vi "FTW-CodeGen-GenerateCode.vi"(0 "State In":T2, 5 "XRef":refnum<vi>, 7 "Terms":T1(array[cluster]), 9 "Diagram":refnum<vi>) -> (4 "State Out":T2, 6 "Reply":string[](array[string]), 8 "Generated Code?":bool)   [LabVIEW 2013, in "Featherweight.lvlib" / "FTW-SQLite-Fetch.xnode"]
uses:
  FTW-SQLite-Fetch.xnode
  FTW-CodeGen-State.ctl
  FTW-CodeGen.lvlib
  Featherweight.lvlib
panel:
  # "Inputs"
  # "Outputs"
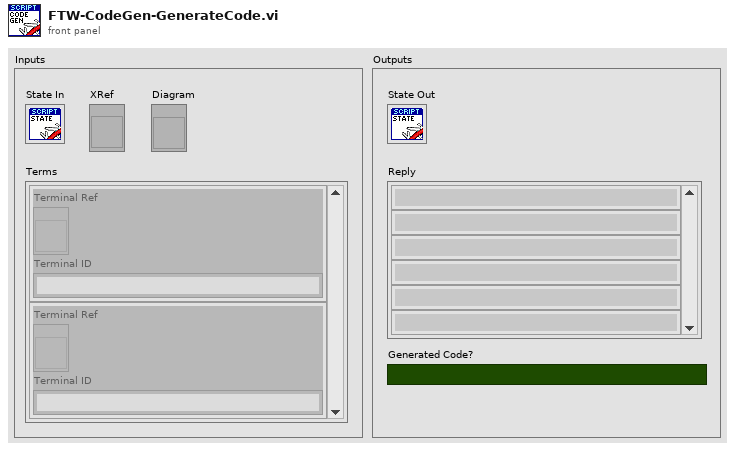
[diagram p1: front panel]
types:
  T1 = cluster{"Terminal Ref":refnum<vi>, "Terminal ID":string}[]
  T2 = typedef "Featherweight.lvlib/FTW-SQLite-Fetch.xnode/FTW-CodeGen-State.ctl" = cluster{"Dummy":string}
  T3 = typedef "LVPositionTypeDef.ctl" = cluster{"Left":i32, "Top":i32}
  T4 = typedef "Featherweight.lvlib/FTW-Reflection-Types.ctl" = enum16{"Unknown", "Void", "Array", "Cluster", "LVObject", "Boolean", "I8", "I16", "I32", "I64", "U8", "U16", "U32", "U64", "SGL", "DBL", "EXT", "CSG", "CDB", "CXT", "FXP", "EnumU8", "EnumU16", "EnumU32", "EnumU64", "SGLwithUnit", "DBLwithUnit", "EXTwithUnit", "CSGwithUnit", "CDBwithUnit", "CXTwithUnit", "String", "Path", "Picture", "Tag", "LVVariant", "Timestamp", "WaveformI8", "WaveformI16", "WaveformI32", "WaveformI64", "WaveformU8", "WaveformU16", "WaveformU32", "WaveformU64", "WaveformSGL", "WaveformDBL", "WaveformEXT", "WaveformCSG", "WaveformCDB", "WaveformCXT", "WaveformDigital", "WaveformUnknownType", "DigitalData", "DynamicData", "ExternalData", "FileByteStream", "TDMStream", "dotNET", "ActiveX", "VIServerReference", "VIReference", "ApplicationInstance", "Menu", "ConnectionDataSocket", "ConnectionVISA", "ConnectionBluetooth", "ConnectionIrDA", "ConnectionTCP", "ConnectionUDP", "ConnectionHTTPClient", "ConnectionFTP", "Occurrence", "Notifier", "Queue", "Rendezvous", "Semaphore", "RTFIFO", "EventPublisher", "EventRegistration", "EventCallback", "DataValueReference", "GenericClass", "GenericClassTag", "GenericClassDeepCopy", "GenericClassFlattened", "GenericClassTagFlattened", "GenericReferenceType", "WindowsRegistry", "OverloadedDatalogRef", "ReferenceUnknownType"}
  T5 = cluster{"Element Name":string, "Element Type":T4, "Element Value":variant}[]
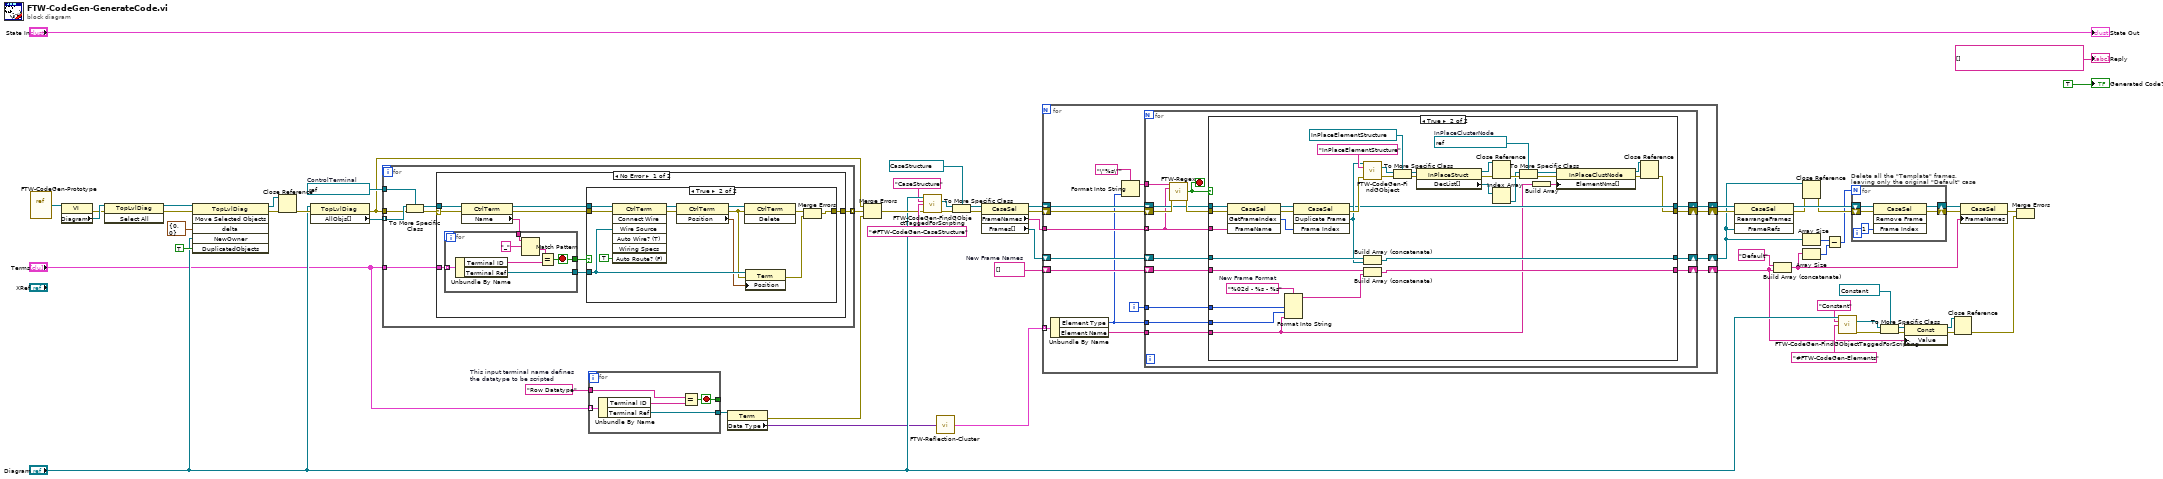
[diagram p0: block diagram]
diagram:
  w19 = string[] []  # New Frame Names
  w38 = "Row Datatype"  # This input terminal name defines the datatype to be scripted
  w57 = refnum<vi> refnum  # ControlTerminal
  n1 = vi-ref "FTW-CodeGen-Prototype.vi"() -> (w50:refnum<vi>)
  n2 = property class="VI"(reference=w50) -> (error out=w49:errorcluster, "Diagram"=w56:refnum<vi>)  [unwired: 1 in, 1 out]
  n3 = invoke class="TopLvlDiag" method="Select All"(reference=w56, error in=w49) -> (reference out=w60:refnum<vi>, error out=w59:errorcluster)  [unwired: 1 in, 1 out]
  n4 = invoke class="TopLvlDiag" method="Move Selected Objects"(reference=w60, error in=w59, "delta"=cluster{"X":i32, "Y":i32} {"X"=0, "Y"=0} ("X/Y Delta"), "NewOwner"="Diagram", "DuplicatedObjects"=TRUE ("Duplicate? (F)")) -> (reference out=w46:refnum<vi>, error out=w48:errorcluster)  [unwired: 1 in, 4 out]
  n5 = Close Reference(reference=w46, error in (no error)=w48) -> (error out=w47:errorcluster)
  n6 = property class="TopLvlDiag"(reference="Diagram", error in=w47) -> (error out=w54:errorcluster, "AllObjs[]"=w58:refnum<vi>[])  [unwired: 1 out]
  n7 = for {
    tunnel: w58 -> [w69] mode=indexing
    tunnel: w54 -> [w68]
    tunnel: w57 -> [w67]
    tunnel: "Terms" -> [w64]
    tunnel: [w63] -> w55 mode=indexing
    n8 = To More Specific Class(target class=w67, reference=w69, error in=w68) -> (specific class reference=w65:refnum<vi>, error out=w66:errorcluster)
    n9 = case shown="No Error" w66 {
      selector: w66 -> [w77 _]
      tunnel: w65 -> [w78 _]
      tunnel: w64 -> [w76 _]
      tunnel: [w71 _] -> w63
      frame No Error {
        n10 = property class="CtrlTerm"(reference=w78, error in=w77) -> (reference out=w73:refnum<vi>, error out=w72:errorcluster, "Name"=w75:string)
        n11 = for {
          tunnel: w76 -> [w98] mode=indexing
          tunnel: w75 -> [w96]
          tunnel: [w97] -> w74
          tunnel: [w92] -> w70
          stop <- w92 stop-if-true
          n12 = Unbundle By Name(w98) -> ("Terminal ID"=w93:string, "Terminal Ref"=w97:refnum<vi>)
          n13 = Match Pattern(string=w96, regular expression="_") -> (after substring=w94:string)  [unwired: 1 in, 3 out]
          n14 = Equal?(x=w94, y=w93) -> (x = y?=w92:bool)
        }
        n15 = case shown="True" w70 {
          tunnel: w74 -> [_ w83]
          tunnel: w73 -> [_ w91]
          tunnel: w72 -> [w79 w90]
          tunnel: [w79 w85] -> w71
          frame False {
          }
          frame True {
            n16 = invoke class="CtrlTerm" method="Connect Wire"(reference=w91, error in=w90, "Wire Source"=w83, "Auto Route? (F)"=TRUE) -> (reference out=w89:refnum<vi>, error out=w87:errorcluster)  [unwired: 3 in, 5 out]
            n17 = property class="CtrlTerm"(reference=w89, error in=w87) -> (reference out=w88:refnum<vi>, error out=w82:errorcluster, "Position"=w80:T3)
            n18 = invoke class="CtrlTerm" method="Delete"(reference=w88, error in=w82) -> (error out=w86:errorcluster)  [unwired: 1 in, 2 out]
            n19 = property class="Term"(reference=w83, error in=w82, "Position"=w80) -> (error out=w81:errorcluster)  [unwired: 1 out]
            n20 = Merge Errors(w86, w81) -> (w85:errorcluster)
          }
        }
      }
      frame Error {
      }
    }
  }
  n21 = for {
    tunnel: "Terms" -> [w103] mode=indexing
    tunnel: [w102] -> w31
    tunnel: [w100] -> _
    tunnel: w38 -> [w99]
    stop <- w100 stop-if-true
    n22 = Unbundle By Name(w103) -> ("Terminal ID"=w101:string, "Terminal Ref"=w102:refnum<vi>)
    n23 = Equal?(x=w99, y=w101) -> (x = y?=w100:bool)
  }
  n24 = property class="Term"(reference=w31) -> (error out=w29:errorcluster, "Data Type"=w30:variant)  [unwired: 1 in, 1 out]
  n25 = Merge Errors(w54, w55, w29) -> (w43:errorcluster)
  n26 = call "FTW-CodeGen-FindGObjectTaggedForScripting.vi"("GObject to Traverse"="Diagram", "Class Name"="CaseStructure", "Label to uniquely identify node"="#FTW-CodeGen-CaseStructure", "error in"=w43) -> ("GObject"=w42:refnum<vi>, "error out"=w41:errorcluster)  [unwired: 10 in]
  n27 = call "FTW-Reflection-Cluster.vi"("Cluster"=w30) -> ("Cluster Elements"=w28:T5)  [unwired: 14 in]
  n28 = To More Specific Class(target class=refnum<vi> refnum ("Object"), reference=w42, error in=w41) -> (specific class reference=w27:refnum<vi>, error out=w25:errorcluster)
  n29 = property class="CaseSel"(reference=w27, error in=w25) -> (reference out=w26:refnum<vi>, error out=w24:errorcluster, "FrameNames"=w23:string[], "Frames[]"=w10:refnum<vi>[])
  n30 = for {
    tunnel: w28 -> [w115] mode=indexing
    tunnel: w23 -> [w116]
    shift-right: [w110] -> w15
    shift-left: w26 -> [w118]
    shift-right: [w111] -> w13
    shift-left: w24 -> [w117]
    shift-right: [w109] -> w9
    shift-left: w10 -> [w112]
    shift-right: [w107] -> w16
    shift-left: w19 -> [w108]
    i -> [w104]
    n31 = Unbundle By Name(w115) -> ("Element Type"=w105:T4, "Element Name"=w106:string)
    n32 = Format Into String(format string="\"%s\"", w105) -> (resulting string=w113:string)  [unwired: 2 in, 1 out]
    n33 = for {
      tunnel: w116 -> [w122] mode=indexing
      tunnel: w113 -> [w132]
      shift-right: [w126] -> w110
      shift-left: w118 -> [w130]
      shift-right: [w128] -> w109
      shift-left: w112 -> [w129]
      shift-right: [w127] -> w111
      shift-left: w117 -> [w133]
      shift-right: [w123] -> w107
      shift-left: w108 -> [w124]
      tunnel: w106 -> [w121]
      tunnel: w105 -> [w120]
      tunnel: w104 -> [w119]
      stop <- w125 stop-if-true
      n34 = call "FTW-Regex.vi"("Regular Expression"=w132, "Input String"=w122, "error in"=w133) -> ("Match Found?"=w125:bool, "error out"=w131:errorcluster)  [unwired: 8 in, 3 out]
      n35 = case shown="True" w125 {
        tunnel: w131 -> [w136 w168]
        tunnel: w130 -> [w137 w169]
        tunnel: w129 -> [w135 w173]
        tunnel: [w135 w170] -> w128
        tunnel: [w136 w144] -> w127
        tunnel: [w137 w148] -> w126
        tunnel: w124 -> [w134 w172]
        tunnel: [w134 w171] -> w123
        tunnel: w122 -> [_ w164]
        tunnel: w121 -> [_ w140]
        tunnel: w120 -> [_ w139]
        tunnel: w119 -> [_ w138]
        frame False {
        }
        frame True {
          w141 = "%02d - %s - %s"  # New Frame Format
          w159 = refnum<vi> refnum  # InPlaceClusterNode
          n36 = invoke class="CaseSel" method="GetFrameIndex"(reference=w169, error in=w168, "FrameName"=w164) -> (reference out=w167:refnum<vi>, error out=w166:errorcluster, "GetFrameIndex"=w165:i32)  [unwired: 1 in, 1 out]
          n37 = Format Into String(format string=w141, w138, w139, w140) -> (resulting string=w142:string)  [unwired: 2 in, 1 out]
          n38 = invoke class="CaseSel" method="Duplicate Frame"(reference=w167, error in=w166, "Frame Index"=w165) -> (reference out=w148:refnum<vi>, error out=w150:errorcluster, "Duplicate Frame"=w149:refnum<vi>)  [unwired: 1 in, 1 out]
          n39 = call "FTW-CodeGen-FindGObject.vi"("GObject to Traverse"=w149, "Class Name"="InPlaceElementStructure", "error in"=w150) -> ("GObject"=w152:refnum<vi>, "error out"=w153:errorcluster)  [unwired: 11 in]
          n40 = Build Array (concatenate)(w173, w149) -> (w170:refnum<vi>[])
          n41 = Build Array (concatenate)(w172, w142) -> (w171:string[])
          n42 = To More Specific Class(target class=refnum<vi> refnum ("Object"), reference=w152, error in=w153) -> (specific class reference=w156:refnum<vi>, error out=w155:errorcluster)
          n43 = property class="InPlaceStruct"(reference=w156, error in=w155) -> (reference out=w162:refnum<vi>, error out=w161:errorcluster, "DecList[]"=w157:refnum<vi>[])
          n44 = Close Reference(reference=w162, error in (no error)=w161) -> (error out=w163:errorcluster)
          n45 = Index Array(array=w157) -> (element=w158:refnum<vi>)  [unwired: 1 in]
          n46 = To More Specific Class(target class=w159, reference=w158, error in=w163) -> (specific class reference=w160:refnum<vi>, error out=w147:errorcluster)
          n47 = Build Array(w140) -> (w143:string[])
          n48 = property class="InPlaceClustNode"(reference=w160, error in=w147, "ElementNms[]"=w143) -> (reference out=w146:refnum<vi>, error out=w145:errorcluster)
          n49 = Close Reference(reference=w146, error in (no error)=w145) -> (error out=w144:errorcluster)
        }
      }
    }
  }
  n50 = invoke class="CaseSel" method="RearrangeFrames"(reference=w15, error in=w13, "FrameRefs"=w9) -> (reference out=w14:refnum<vi>, error out=w12:errorcluster)  [unwired: 1 in, 2 out]
  n51 = Build Array (concatenate)("Default", w16) -> (w8:string[])
  n52 = Close Reference(reference=w9, error in (no error)=w12) -> (error out=w11:errorcluster)
  n53 = Array Size(array=w9) -> (size(s)=w7:i32)
  n54 = Array Size(array=w8) -> (size(s)=w6:i32)
  n55 = Subtract(x=w7, y=w6) -> (x-y=w5:i32)
  n56 = call "FTW-CodeGen-FindGObjectTaggedForScripting.vi"("GObject to Traverse"="Diagram", "Class Name"="Constant", "Label to uniquely identify node"="#FTW-CodeGen-Elements") -> ("GObject"=w35:refnum<vi>, "error out"=w34:errorcluster)  [unwired: 11 in]
  n57 = for "Delete all the \"Template\" frames,\nleaving only the original \"Default\" case" {
    N: w5 -> [_]
    shift-right: [w175] -> w21
    shift-left: w11 -> [w176]
    shift-right: [w177] -> w22
    shift-left: w14 -> [w178]
    n58 = invoke class="CaseSel" method="Remove Frame"(reference=w178, error in=w176, "Frame Index"=u32 1) -> (reference out=w177:refnum<vi>, error out=w175:errorcluster)  [unwired: 1 in, 2 out]
  }
  n59 = To More Specific Class(target class=refnum<vi> refnum ("Object"), reference=w35, error in=w34) -> (specific class reference=w33:refnum<vi>, error out=w32:errorcluster)
  n60 = property class="Const"(reference=w33, error in=w32, "Value"=w16) -> (reference out=w4:refnum<vi>, error out=w3:errorcluster)
  n61 = Close Reference(reference=w4, error in (no error)=w3) -> (error out=w1:errorcluster)
  n62 = property class="CaseSel"(reference=w22, error in=w21, "FrameNames"=w8) -> (error out=w2:errorcluster)  [unwired: 1 out]
  n63 = Merge Errors(w2, w1) -> ()  [unwired: 1 out]
  "State Out" <- "State In"
  "Reply" <- string[] [] ("Reply")
  "Generated Code?" <- TRUE ("Generated Code?")
